vi "Labels Change and Make Unique.vi"(1 "Force Update":bool, 2 "Labels":string[](array[string]), 3 "Configured Inst Input":T1[](array[typedef]) {"Private"."Offset" format="%^_3e"; "Private"."Scale Factors" format="%^_3e"}) -> (0 "Configured Inst dup":T1[](array[typedef]) {"Private"."Offset" format="%^_3e"; "Private"."Scale Factors" format="%^_3e"})   [LabVIEW 2020]
uses:
  Sub Controls/Instrument Properties.ctl
  Sub Controls/Public.ctl
  Sub Controls/Private.ctl
  Sub Controls/Instrument Ref.ctl
  Sub Controls/SystemCheckBox-resize.ctl
  <vilib>/regexp/Match Regular Expression.xnode
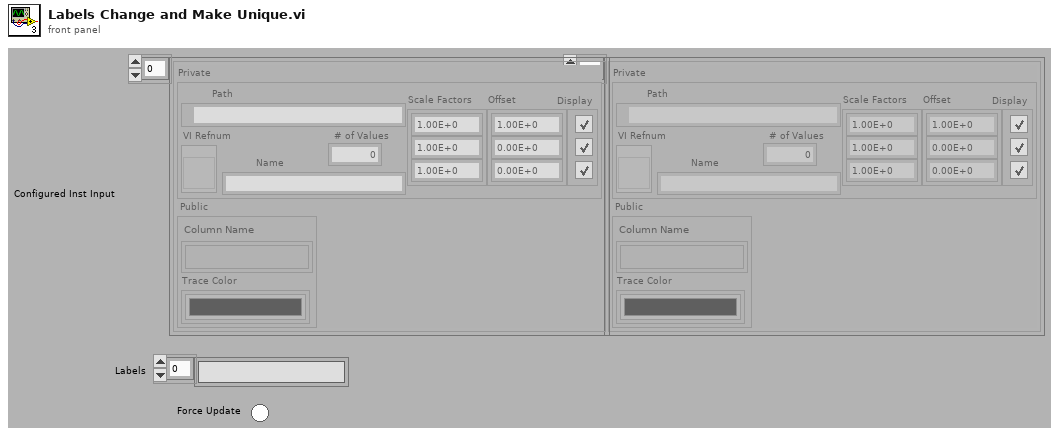
[diagram p1: front panel]
types:
  T1 = typedef "Instrument Properties.ctl" = cluster{"Public":T2, "Private":T3}
  T2 = typedef "Public.ctl" = cluster{"Column Name":string[], "Trace Color":u32[]}
  T3 = typedef "Private.ctl" = cluster{"Path":path, "VI Refnum":T4, "Name":string, "# of Values":i32, "Scale Factors":dbl[], "Display":T5[], "Offset":dbl[]}
  T4 = typedef "Instrument Ref.ctl" = refnum<vi>
  T5 = typedef "SystemCheckBox-resize.ctl" = bool
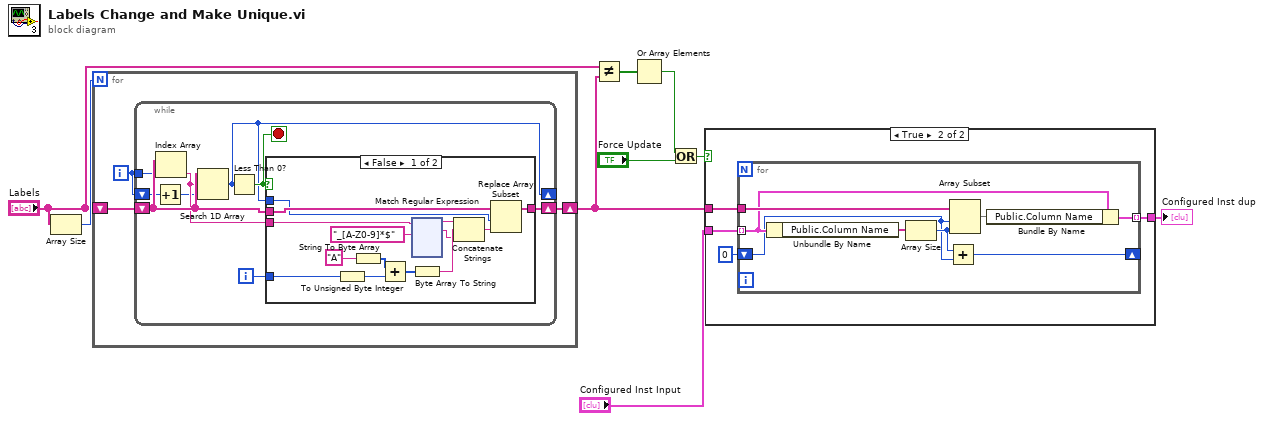
[diagram p0: block diagram]
diagram:
  n1 = Array Size(array="Labels") -> (size(s)=w6:i32)
  n2 = for {
    N: w6 -> [_]
    shift-right: [w11] -> w4
    shift-left: "Labels" -> [w12]
    i -> [w10]
    n3 = while {
      shift-right: [w13] -> _
      shift-left: w10 -> [w14]
      shift-right: [w19] -> w11
      shift-left: w12 -> [w20]
      tunnel: w10 -> [w15]
      i -> [w17]
      stop <- w21 stop-if-true
      n4 = Increment(x=w14) -> (x+1=w16:i32)
      n5 = Index Array(array=w20, index=w15) -> (element=w18:string)
      n6 = Search 1D Array(1D array=w20, element=w18, start index (0)=w16) -> (index of element=w13:i32)
      n7 = Less Than 0?(x=w13) -> (x < 0?=w21:bool)
      n8 = case shown="False" w21 {
        tunnel: w13 -> [w33 _]
        tunnel: w20 -> [w34 w147]
        tunnel: [w35 w147] -> w19
        tunnel: w18 -> [w23 _]
        tunnel: w17 -> [w29 _]
        frame False {
          n9 = To Unsigned Byte Integer(number=w29) -> (unsigned 8bit integer=w28:u8)
          n10 = String To Byte Array(string="A") -> (unsigned byte array=w31:u8[])
          n11 = Add(x=w31, y=w28) -> (x+y=w32:u8[])
          n12 = xnode "Match Regular Expression"("input string"=w23, "regular expression"="_[A-Z0-9]*$") -> ("before match"=w25:string, "whole match"=w24:string)  [unwired: 4 in, 3 out]
          n13 = Byte Array To String(unsigned byte array=w32) -> (string=w27:string)
          n14 = Concatenate Strings(w25, w27, w24) -> (w26:string)
          n15 = Replace Array Subset(array=w34, new element=w26, index=w33) -> (w35:string[])
        }
        frame True {
        }
      }
    }
  }
  n16 = Not Equal?(x="Labels", y=w4) -> (x != y?=w7:bool[])
  n17 = Or Array Elements(Boolean array=w7) -> (logical OR=w3:bool)
  n18 = Or(x=w3, y="Force Update") -> (x .or. y?=w2:bool)
  n19 = case shown="True" w2 {
    tunnel: "Configured Inst Input" -> [w148 w152]
    tunnel: [w148 w149] -> w9
    tunnel: w4 -> [_ w150]
    frame False {
    }
    frame True {
      n20 = for {
        tunnel: w152 -> [w157] mode=indexing
        shift-right: [w159] -> _
        shift-left: 0 -> [w153]
        tunnel: w150 -> [w158]
        tunnel: [w156] -> w149 mode=indexing
        n21 = Unbundle By Name(w157) -> ("Public.Column Name"=w160:string[])
        n22 = Array Size(array=w160) -> (size(s)=w154:i32)
        n23 = Add(x=w154, y=w153) -> (x+y=w159:i32)
        n24 = Array Subset(array=w158, index=w153, length=w154) -> (w155:string[])
        n25 = Bundle By Name(cluster=w157, "Public.Column Name"=w155) -> (w156:T1)
      }
    }
  }
  "Configured Inst dup" <- w9
